vi "Initialize KUKA youBot.vi"(8 "error in (no error)":errorcluster) -> (0 "error out":errorcluster, 3 "KUKA youBot host out":refnum<class "NI_Robotics_KUKA youBot Host_EtherCAT.lvclass">)   [LabVIEW 2017, in "NI_Robotics_KUKA youBot Host.lvlib" / "NI_Robotics_KUKA youBot Host_EtherCAT.lvclass"]
doc: "Initializes an EtherCAT host interface to a real KUKA youBot."
uses:
  <vilib>/robotics/KUKA youBot/EtherCAT Host Interface/NI_Robotics_KUKA youBot Host_EtherCAT.lvclass
  c:/Program Files (x86)/National Instruments/LabVIEW 2017/vi.lib/robotics/KUKA youBot/Host Interface/NI_Robotics_KUKA youBot Host Interface.lvclass
  <vilib>/robotics/KUKA youBot/Host Interface/NI_Robotics_KUKA youBot Host Interface.lvclass/NI_Robotics_KUKA youBot Host Interface.ctl
  <vilib>/robotics/KUKA youBot/Basic Device/Mobile Platform EtherCAT/NI_Robotics_KUKA youBot Platform_EtherCAT.lvclass
  c:/Program Files (x86)/National Instruments/LabVIEW 2017/vi.lib/robotics/KUKA youBot/Basic Device/Mobile Platform/NI_Robotics_KUKA youBot Platform.lvclass
  <vilib>/robotics/KUKA youBot/Basic Device/Arm EtherCAT/NI_Robotics_KUKA youBot Arm_EtherCAT.lvclass
  c:/Program Files (x86)/National Instruments/LabVIEW 2017/vi.lib/robotics/KUKA youBot/Basic Device/Arm/NI_Robotics_KUKA youBot Arm.lvclass
  <resource>/objmgr/IndComECAT.rc
  <vilib>/robotics/KUKA youBot/NI_Robotics_KUKA youBot Host.lvlib
  <vilib>/robotics/KUKA youBot/Host Interface/NI_Robotics_KUKA youBot Host Interface.lvclass
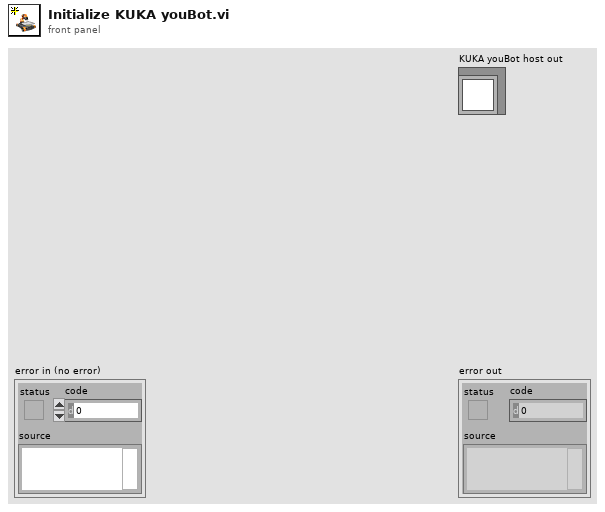
[diagram p1: front panel]
types:
  T1 = typedef "NI_Robotics_KUKA youBot Host.lvlib/Motor Slave Info.ctl" = cluster{"controller mode var":refnum<k21>, "reference var":refnum<k21>, "current var":refnum<k21>, "velocity var":refnum<k21>, "position var":refnum<k21>, "status var":refnum<k21>, "valid":bool, "status var type":enum16{"Int16", "Int32"}, "nodeAddr":u16, "masterHdl":T2}
  T2 = typedef "NI_Robotics_KUKA youBot Host.lvlib/Mater Handler.ctl" = i32
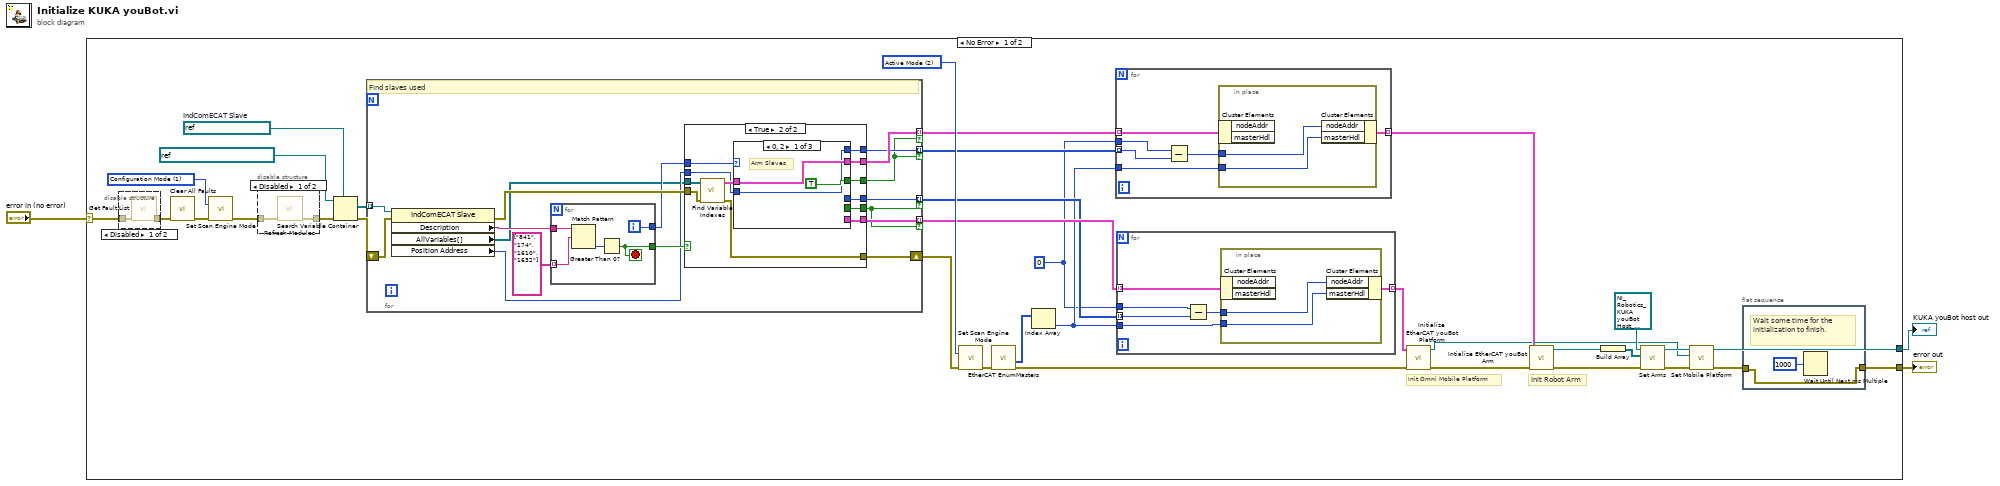
[diagram p0: block diagram]
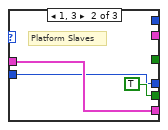
[diagram p5: hidden frame]
diagram:
  n1 = case shown="No Error" "error in (no error)" {
    selector: "error in (no error)" -> [w25 w102]
    tunnel: [w4 w102] -> w2
    tunnel: [w28 _] -> w1
    frame No Error {
      w9 = i16 0
      w18 = 2 items=["Configuration Mode"=1, "Active Mode"=2] ("mode (Active Mode)")
      w32 = refnum<k21> refnum  # IndComECAT Slave
      w37 = 1 items=["Configuration Mode"=1, "Active Mode"=2] ("mode (Active Mode)")
      # "Init Robot Arm"
      # "Init Omni Mobile Platform"
      n2 = disable-structure shown="Disabled" {
        disable-tunnel: [w39 w40] -> w33
        disable-tunnel: w25 -> [w38 w40]
        frame Disabled {
          n3 = call <vilib>:"Get Fault List.vi"("error in (no error)"=w38) -> ("error out"=w39:errorcluster)  [unwired: 9 in, 1 out]
        }
        frame Enabled {
        }
      }
      n4 = call <vilib>:"Clear All Faults.vi"("error in (no error)"=w33) -> ("error out"=w36:errorcluster)  [unwired: 10 in]
      n5 = call <vilib>:"Set Scan Engine Mode.vi"("mode (Active Mode)"=w37, "error in (no error)"=w36) -> ("error out"=w35:errorcluster)  [unwired: 13 in]
      n6 = disable-structure shown="Disabled" {
        disable-tunnel: w35 -> [w42 w43]
        disable-tunnel: [w41 w43] -> w34
        frame Disabled {
          n7 = call <vilib>:"Refresh Modules.vi"("error in (no error)"=w42) -> ("error out"=w41:errorcluster)  [unwired: 10 in]
        }
        frame Enabled {
        }
      }
      n8 = Search Variable Container(7:w32, 8:w34, 11:refnum<k21> "ni.var.io:" ("container refnum in")) -> (0:w29:errorcluster, 2:w30:refnum<k21>[])  [unwired: 3 in, 1 out]
      n9 = for {
        tunnel: w30 -> [w77] mode=indexing
        shift-right: [w72] -> w27
        shift-left: w29 -> [w76]
        tunnel: [w71] -> w16 mode=indexing if=w66
        tunnel: [w68] -> w17 mode=indexing if=w64
        tunnel: [w67] -> w15 mode=indexing if=w66
        tunnel: [w65] -> w14 mode=indexing if=w64
        # "Find slaves used"
        n10 = property class="IndComECAT Slave"(reference=w77, error in=w76) -> (error out=w73:errorcluster, "Description"=w74:string, "AllVariables[]"=w62:refnum<k21>[], "Position Address"=w63:u16)  [unwired: 1 out]
        n11 = for {
          tunnel: string[] ["841", "174", "1610", "1632"] -> [w100] mode=indexing
          tunnel: [w99] -> w70
          tunnel: w74 -> [w98]
          tunnel: [w97] -> w69
          i -> [w97]
          stop <- w99 stop-if-true
          n12 = Match Pattern(string=w98, regular expression=w100) -> (offset past match=w101:i32)  [unwired: 1 in, 3 out]
          n13 = Greater Than 0?(x=w101) -> (x > 0?=w99:bool)
        }
        n14 = case shown="True" w70 {
          tunnel: w62 -> [_ w90]
          tunnel: w73 -> [w78 w89]
          tunnel: [w78 w88] -> w72
          tunnel: [_ w85] -> w71
          tunnel: w69 -> [_ w87]
          tunnel: w63 -> [_ w84]
          tunnel: [_ w83] -> w66
          tunnel: [_ w82] -> w68
          tunnel: [_ w81] -> w64
          tunnel: [_ w80] -> w67
          tunnel: [_ w79] -> w65
          frame False {
          }
          frame True {
            n15 = call <vilib>:"Find Variable Indexes.vi"("error in (no error)"=w89, "all variables"=w90) -> ("error out"=w88:errorcluster, "motor slave info"=w86:T1)  [unwired: 7 in, 1 out]
            n16 = case shown="0, 2" w87 {
              tunnel: w86 -> [w92 w95 _]
              tunnel: [w92 _ _] -> w85
              tunnel: w84 -> [w91 w94 _]
              tunnel: [TRUE _ _] -> w83
              tunnel: [_ w95 _] -> w82
              tunnel: [_ TRUE _] -> w81
              tunnel: [w91 _ _] -> w80
              tunnel: [_ w94 _] -> w79
              frame 0, 2 {
                # "Arm Slaves"
              }
              frame 1, 3 {
                # "Platform Slaves"
              }
              frame Default {
              }
            }
          }
        }
      }
      n17 = call <vilib>:"Set Scan Engine Mode.vi"("mode (Active Mode)"=w18, "error in (no error)"=w27) -> ("error out"=w21:errorcluster)  [unwired: 13 in]
      n18 = call <vilib>:"EtherCAT EnumMasters.vi"("error in (no error)"=w21) -> ("error out"=w11:errorcluster, "masterHdls"=w10:T2[])  [unwired: 9 in]
      n19 = Index Array(array=w10) -> (element=w12:T2)  [unwired: 1 in]
      n20 = for {
        tunnel: [w51] -> w26 mode=indexing
        tunnel: w12 -> [w50]
        tunnel: w16 -> [w49] mode=indexing
        tunnel: w15 -> [w46] mode=indexing
        tunnel: w9 -> [w47]
        n21 = Subtract(x=w47, y=w46) -> (x-y=w48:u16)
        n22 = in-place {
          in-place-border: w50 -> [w53]
          in-place-border: w48 -> [w52]
          n23 = in-place-cluster #1(w49) -> ()  [unwired: 2 out]
          n24 = in-place-cluster #1("nodeAddr"=w52, "masterHdl"=w53) -> (w51:T1)
        }
      }
      n25 = for {
        tunnel: [w59] -> w13 mode=indexing
        tunnel: w12 -> [w58]
        tunnel: w17 -> [w57] mode=indexing
        tunnel: w9 -> [w56]
        tunnel: w14 -> [w55] mode=indexing
        n26 = Subtract(x=w56, y=w55) -> (x-y=w54:u16)
        n27 = in-place {
          in-place-border: w58 -> [w61]
          in-place-border: w54 -> [w60]
          n28 = in-place-cluster #2(w57) -> ()  [unwired: 2 out]
          n29 = in-place-cluster #2("nodeAddr"=w60, "masterHdl"=w61) -> (w59:T1)
        }
      }
      n30 = call <vilib>:"Initialize EtherCAT youBot Platform.vi"("error in (no error)"=w11, "arm slave infos"=w13) -> ("error out"=w19:errorcluster, "KUKA youBot platform_EtherCAT out"=w20:refnum<class "NI_Robotics_KUKA youBot Platform_EtherCAT.lvclass">)  [unwired: 8 in]
      n31 = call <vilib>:"Intialize EtherCAT youBot Arm.vi"("error in (no error)"=w19, "arm slave infos"=w26) -> ("error out"=w8:errorcluster, "KUKA youBot arm_EtherCAT out"=w7:refnum<class "NI_Robotics_KUKA youBot Arm_EtherCAT.lvclass">)  [unwired: 8 in]
      n32 = Build Array(w7) -> (w6:refnum<class "NI_Robotics_KUKA youBot Arm_EtherCAT.lvclass">[])
      n33 = call <vilib>:"Set Arms.vi"("error in (no error)"=w8, "arms"=w6, "KUKA youBot host in"=refnum<class "NI_Robotics_KUKA youBot Host_EtherCAT.lvclass"> refnum ("NI_Robotics_KUKA youBot Host.lvlib:NI_Robotics_KUKA youBot Host_EtherCAT.lvclass")) -> ("error out"=w24:errorcluster, "KUKA youBot host out"=w22:refnum<class "NI_Robotics_KUKA youBot Host_EtherCAT.lvclass">)  [unwired: 7 in]
      n34 = call <vilib>:"Set Mobile Platform.vi"("error in (no error)"=w24, "KUKA youBot platform in"=w20, "KUKA youBot host in"=w22) -> ("error out"=w5:errorcluster, "KUKA youBot host out"=w28:refnum<class "NI_Robotics_KUKA youBot Host_EtherCAT.lvclass">)  [unwired: 7 in]
      n35 = flat-sequence {
        tunnel: w5 -> [w44]
        tunnel: [w44] -> w4
        frame #0 {
          # "Wait some time for the initialization to finish."
          n36 = Wait Until Next ms Multiple(millisecond multiple=u32 1000) -> ()  [unwired: 1 out]
        }
      }
    }
    frame Error {
    }
  }
  "error out" <- w2
  "KUKA youBot host out" <- w1
